vi "VI_ChList_ParseStringList.vi"(8 "error in (no error)":errorcluster, 11 "ChList_RawString":string) -> (0 "error out":errorcluster, 3 "Channel List":cluster{"ID":string, "Name":string}[](array[cluster]))   [LabVIEW 2020, in "OXYGEN_Datastream.lvlib"]
uses:
  OXYGEN_Datastream.lvlib
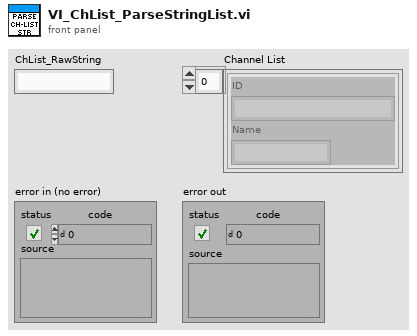
[diagram p1: front panel]
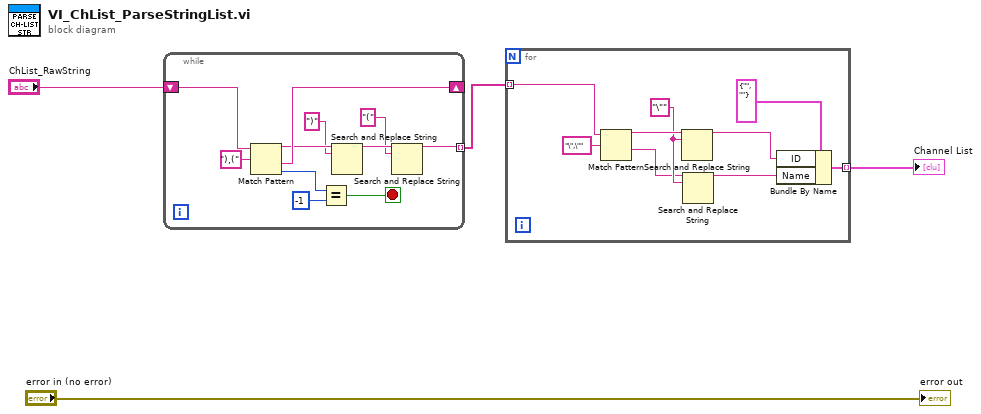
[diagram p0: block diagram]
diagram:
  n1 = while {
    shift-right: [w10] -> _
    shift-left: "ChList_RawString" -> [w12]
    tunnel: [w6] -> w3 mode=indexing
    stop <- w13 stop-if-true
    n2 = Match Pattern(string=w12, regular expression="),(") -> (before substring=w9:string, after substring=w10:string, offset past match=w15:i32)  [unwired: 1 in, 1 out]
    n3 = Equal?(x=w15, y=-1) -> (x = y?=w13:bool)
    n4 = Search and Replace String(input string=w9, search string=")" ("substring (\"\")")) -> (result string=w7:string)  [unwired: 6 in, 3 out]
    n5 = Search and Replace String(input string=w7, search string="(" ("substring (\"\")")) -> (result string=w6:string)  [unwired: 6 in, 3 out]
  }
  n6 = for {
    tunnel: w3 -> [w22] mode=indexing
    tunnel: [w16] -> w2 mode=indexing
    w21 = "\"" ("substring (\"\")")
    n7 = Match Pattern(string=w22, regular expression="\",\"") -> (before substring=w24:string, after substring=w20:string)  [unwired: 1 in, 2 out]
    n8 = Search and Replace String(input string=w24, search string=w21) -> (result string=w18:string)  [unwired: 6 in, 3 out]
    n9 = Search and Replace String(input string=w20, search string=w21) -> (result string=w17:string)  [unwired: 6 in, 3 out]
    n10 = Bundle By Name(cluster=cluster{"ID":string, "Name":string} {"ID"="", "Name"=""} ("ChannelList_Names"), "ID"=w18, "Name"=w17) -> (w16:cluster{"ID":string, "Name":string})
  }
  "Channel List" <- w2
  "error out" <- "error in (no error)"
